vi "SimulatedSignal4.vi"(11 "Phase":fxp<+,64,64>[](array[numeric])=[0.0, 0.0, 0.0, 0.0]) -> (2 "dummy do not use":i16[](array[numeric]), 3 "output":T1)   [LabVIEW 2013]
uses:
  subVIs/I16 array size 4.ctl
  <vilib>/rvi/FXPMathLib/FxpInterpret/XNode/nifxpmath_Interpret.xnode
  <vilib>/rvi/FXPMathLib/FxpSub/XNode/nifxpmath_Sub.xnode
  <vilib>/rvi/FXPMathLib/sim/FxpSim.dll
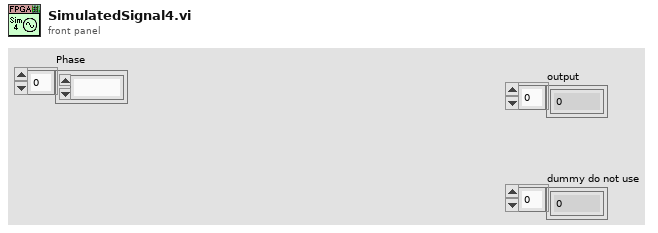
[diagram p1: front panel]
types:
  T1 = typedef "I16 array size 4.ctl" = i16[]
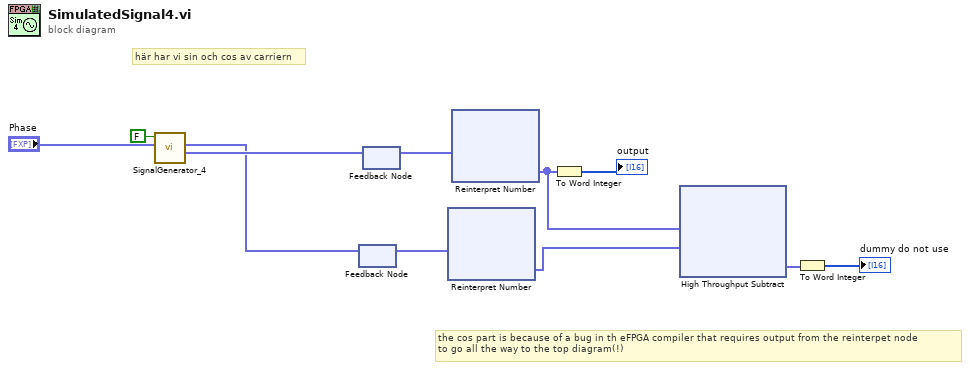
[diagram p0: block diagram]
diagram:
  # "the cos part is because of a bug in th eFPGA compiler that requires output from the reinterpet node\nto go all the way to the top diagram(!)"
  # "här har vi sin och cos av carriern"
  n1 = call "SignalGenerator_4.vi"("Phase"="Phase", "reset"=FALSE) -> ("Sine out"=w3:fxp<+/-,16,0>[], "Cosine out"=w2:fxp<+/-,16,0>[])  [unwired: 8 in]
  n2 = feedback #1() -> (w9:fxp<+/-,16,0>[])  [unwired: 1 in]
  n3 = feedback-in #1(w2) -> ()
  n4 = feedback #2() -> (w11:fxp<+/-,16,0>[])  [unwired: 1 in]
  n5 = feedback-in #2(w3) -> ()
  n6 = xnode "Reinterpret Number"("x"=w9) -> ("y"=w7:fxp<+/-,16,16>[])
  n7 = xnode "Reinterpret Number"("x"=w11) -> ("y"=w8:fxp<+/-,16,16>[])
  n8 = To Word Integer(number=w8) -> (16bit integer=→"output":i16[])
  n9 = xnode ("High Throughput Subtract")("x"=w8, "y"=w7) -> ("x-y"=w6:fxp<+/-,17,17>[])
  n10 = To Word Integer(number=w6) -> (16bit integer=→"dummy do not use":i16[])
